vi "Launch Nested.vi"(8 "Error In":errorcluster, 9 "ID":string, 10 "Nested Actor":refnum<class "Actor.lvclass">, 11 "Controller in":refnum<class "Controller.lvclass">) -> (0 "Error Out":errorcluster, 3 "Controller out":refnum<class "Controller.lvclass">)   [LabVIEW 2014, in "Controller.lvlib" / "Controller.lvclass"]
doc: "This VI launches the nested actor and then stores the enqueuer in a MAP object (represented by variant attributes). The enqueuer name is based on a unique <b>ID</b>. Each time an object is added, the attribute <b>NumActive</b> is incremented, the actual object (Enqueuer) is stored with a key value of <b>ID</b> and the key is added to a list of attributes called <b>IDs</b>. \n\nThe <b>NumActive</b> allows the MAP to indicate when it is empty. This is used when stopping the system.\n\nIf the launch is unsuccessful, the enqueuer is not stored and the MAP is not affected."
uses:
  Controller.lvclass
  <vilib>/ActorFramework/Actor/Actor.lvclass
  Controller.lvclass/Controller.ctl
  Controls/eMap.ctl
  <vilib>/ActorFramework/Message Enqueuer/Message Enqueuer.lvclass
  SuperActor/Ex Nested.lvclass/Ex Nested.ctl
  SuperActor/Read Log Session.vi
  <userlib>/_Session Fwk/Session - Root.lvclass
  reusable/Session APIs/Session Log/System Log.lvclass
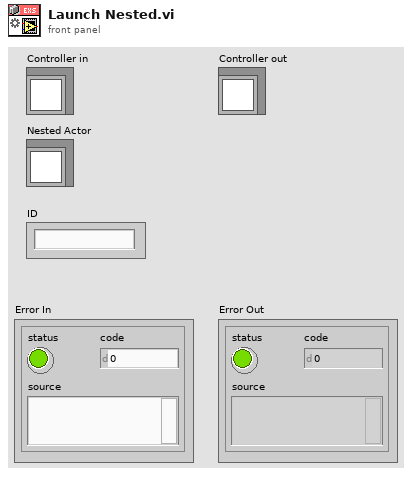
[diagram p1: front panel]
types:
  T1 = typedef "Controller.lvlib/Controller.lvclass/eMap.ctl" = cluster{"Enqueuer":refnum<class "Message Enqueuer.lvclass">, "Active":bool}
  T2 = typedef "Session - Root.lvclass/Session Handle.ctl" = refnum<data-value>
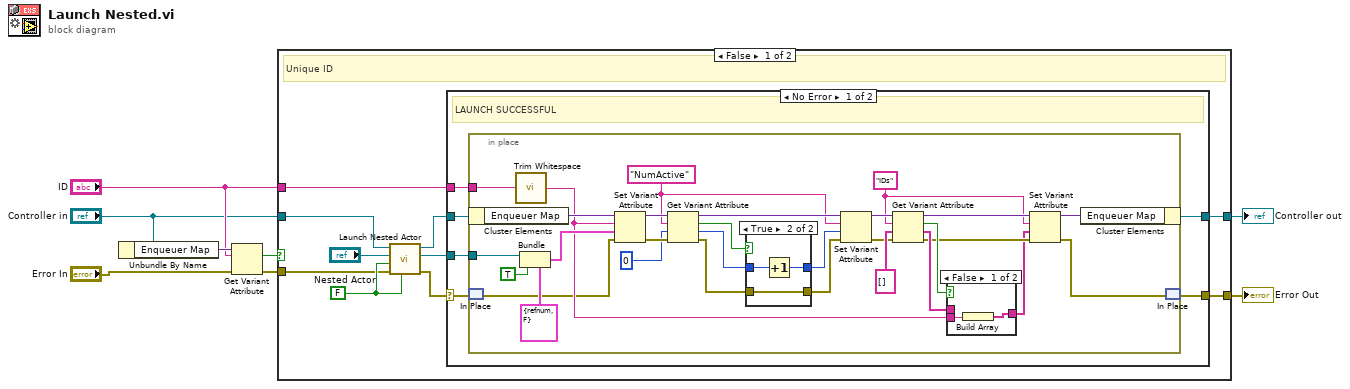
[diagram p0: block diagram]
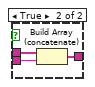
[diagram p2: hidden frame]
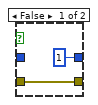
[diagram p3: hidden frame]
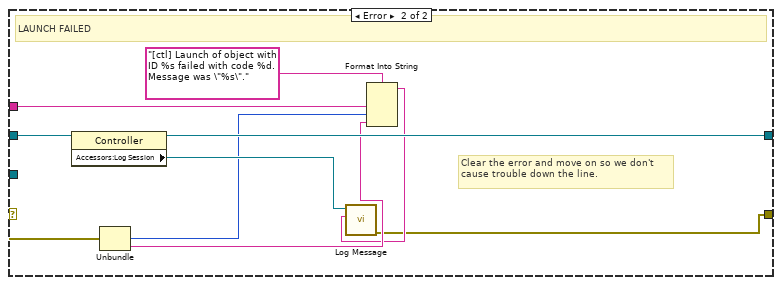
[diagram p4: hidden frame]
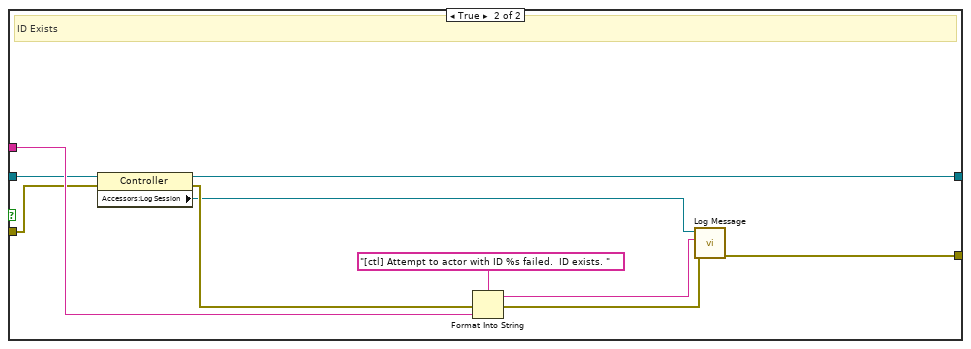
[diagram p5: hidden frame]
diagram:
  n1 = Unbundle By Name("Controller in") -> ("Enqueuer Map"=w8:variant)
  n2 = Get Variant Attribute(Variant=w8, name="ID", error in="Error In") -> (found=w2:bool, error out=w1:errorcluster)  [unwired: 1 in, 2 out]
  n3 = case shown="False" w2 {
    tunnel: "ID" -> [w14 w79]
    tunnel: [w13 w77] -> w5
    tunnel: [w12 w80] -> w4
    tunnel: "Controller in" -> [w11 w78]
    tunnel: w1 -> [w9 w75]
    frame False {
      w16 = FALSE ("Open Actor Core front panel? (F)")
      # "Unique ID"
      n4 = call <vilib>:"Launch Nested Actor.vi"("Open Actor Core front panel? (F)"=w16, "error in (no error)"=w9, "Auto-stop? (T)"=w16, "Nested Actor"="Nested Actor", "Caller Actor in"=w11) -> ("error out"=w17:errorcluster, "Nested Actor's Enqueuer"=w18:refnum<class "Message Enqueuer.lvclass">, "Caller Actor out"=w10:refnum<class "Controller.lvclass">)  [unwired: 4 in]
      n5 = case shown="No Error" w17 {
        selector: w17 -> [w20 w70]
        tunnel: w10 -> [w24 w73]
        tunnel: [w23 w72] -> w13
        tunnel: w18 -> [w22 _]
        tunnel: [w19 w64] -> w12
        tunnel: w14 -> [w21 w68]
        frame No Error {
          # "LAUNCH SUCCESSFUL"
          n6 = in-place {
            in-place-border: w22 -> [w52]
            in-place-border: w21 -> [w28]
            w30 = "IDs" ("name")
            w41 = "NumActive" ("name")
            n7 = in-place-cluster #1(w24) -> ("Enqueuer Map"=w53:variant)
            n8 = in-place-match #2(w20) -> (w26:errorcluster)
            n9 = call <vilib>:"Trim Whitespace.vi"("string"=w28) -> ("trimmed string"=w27:string)  [unwired: 1 in]
            n10 = Bundle(cluster=T1 {"Enqueuer"=refnum, "Active"=FALSE} ("eMap"), "Enqueuer"=w52, "Active"=TRUE) -> (w51:T1)
            n11 = Set Variant Attribute(Variant=w53, name=w27, value=w51, error in=w26) -> (Variant out=w48:variant, error out=w49:errorcluster)  [unwired: 1 out]
            n12 = Get Variant Attribute(Variant=w48, name=w41, default value (empty Variant)=i16 0 ("unsigned 8bit integer"), error in=w49) -> (duplicate Variant=w45:variant, found=w44:bool, value=w47:i16, error out=w43:errorcluster)
            n13 = case shown="True" w44 {
              tunnel: w47 -> [_ w61]
              tunnel: [i16 1 w63] -> w46
              tunnel: w43 -> [w59 w62]
              tunnel: [w59 w62] -> w42
              frame False {
              }
              frame True {
                n14 = Increment(x=w61) -> (x+1=w63:i16)
              }
            }
            n15 = Set Variant Attribute(Variant=w45, name=w41, value=w46, error in=w42) -> (Variant out=w39:variant, error out=w37:errorcluster)  [unwired: 1 out]
            n16 = Get Variant Attribute(Variant=w39, name=w30, default value (empty Variant)=string[] [], error in=w37) -> (duplicate Variant=w34:variant, found=w36:bool, value=w35:string[], error out=w32:errorcluster)
            n17 = case shown="False" w36 {
              tunnel: w35 -> [_ w58]
              tunnel: w27 -> [w55 w57]
              tunnel: [w54 w56] -> w31
              frame False {
                n18 = Build Array(w55) -> (w54:string[])
              }
              frame True {
                n19 = Build Array (concatenate)(w58, w57) -> (w56:string[])
              }
            }
            n20 = Set Variant Attribute(Variant=w34, name=w30, value=w31, error in=w32) -> (Variant out=w33:variant, error out=w25:errorcluster)  [unwired: 1 out]
            n21 = in-place-cluster #1("Enqueuer Map"=w33) -> (w23:refnum<class "Controller.lvclass">)
            n22 = in-place-match #2(w25) -> (w19:errorcluster)
          }
        }
        frame Error {
          # "Clear the error and move on so we don't cause trouble down the line."
          # "LAUNCH FAILED"
          n23 = property class="Controller"(reference=w73) -> (reference out=w72:refnum<class "Controller.lvclass">, "Accessors:Log Session"=w71:T2)  [unwired: 1 in, 1 out]
          n24 = Unbundle(w70) -> ("code"=w67:i32, "source"=w66:string)  [unwired: 1 out]
          n25 = Format Into String(format string="[ctl] Launch of object with ID %s failed with code %d.  Message was \"%s\".", w68, w67, w66) -> (resulting string=w65:string)  [unwired: 2 in, 1 out]
          n26 = call "Log Message.vi"("MSG In"=w65, "session in"=w71) -> ("error out"=w64:errorcluster)  [unwired: 8 in, 1 out]
        }
      }
    }
    frame True {
      # "ID Exists"
      n27 = property class="Controller"(reference=w78, error in=w75) -> (reference out=w77:refnum<class "Controller.lvclass">, error out=w76:errorcluster, "Accessors:Log Session"=w74:T2)
      n28 = Format Into String(format string="[ctl] Attempt to actor with ID %s failed.  ID exists. ", error in=w76, w79) -> (resulting string=w82:string, error out=w81:errorcluster)  [unwired: 1 in]
      n29 = call "Log Message.vi"("error in"=w81, "MSG In"=w82, "session in"=w74) -> ("error out"=w80:errorcluster)  [unwired: 7 in, 1 out]
    }
  }
  "Controller out" <- w5
  "Error Out" <- w4
